vi "Write Event Details.vi"(0 "stop":bool, 1 "OK Button":bool, 2 "Event Details":string, 3 "Event Name":string) -> ()   [LabVIEW 2014]
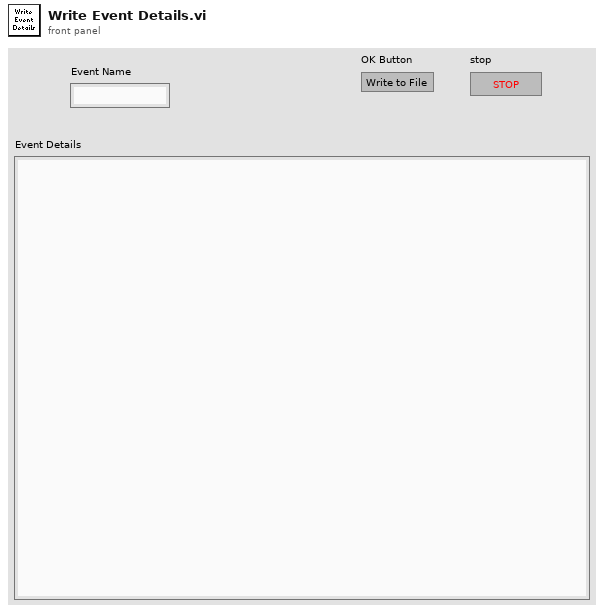
[diagram p1: front panel]
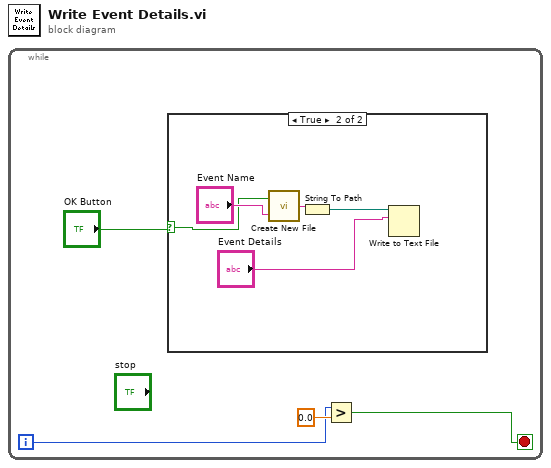
[diagram p0: block diagram]
diagram:
  n1 = while {
    i -> [w2]
    stop <- w1 stop-if-true
    n2 = case shown="True" "OK Button" {
      selector: "OK Button" -> [_ w5]
      frame False {
      }
      frame True {
        n3 = call "Create New File.vi"("Event Name"="Event Name", "OK Button"=w5) -> ("concatenated string"=w7:string)
        n4 = String To Path(string=w7) -> (path=w9:path)
        n5 = Write to Text File(file (use dialog)=w9, text="Event Details") -> ()  [unwired: 2 in, 3 out]
      }
    }
    n6 = Greater?(x=w2, y=0.0) -> (0:w1:bool)
  }
